vi "adder.vi"() -> ()   [LabVIEW 2015]
panel:
  out "x+y":dbl
  in  "x":dbl
  in  "y":dbl
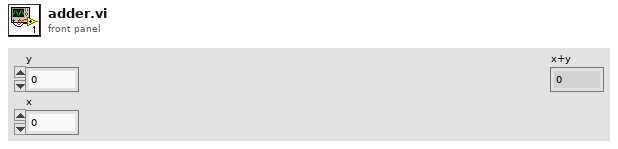
[diagram p1: front panel]
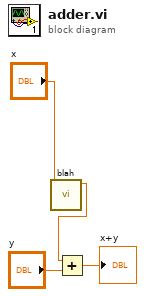
[diagram p0: block diagram]
diagram:
  n1 = call "blah.vi"("x"="x") -> ("Numeric"=w1:dbl)  [unwired: 10 in]
  n2 = Add(x=w1, y="y") -> (x+y=→"x+y":dbl)
